vi "Find Post-Setup Actors.vi"(11 "Base Actor in":refnum<class "Base Actor.lvclass">) -> (2 "Post-Setup Actors":refnum<class "Actor.lvclass">[](array[class]))   [LabVIEW 2020, in "jettl.lvlib" / "Base jettl Actor.lvlib" / "Base Actor.lvlib" / "Base Actor.lvclass"]
uses:
  Base Actor.lvclass
  Base Actor.lvclass/Base Actor.ctl
  Actor/Actor.lvclass
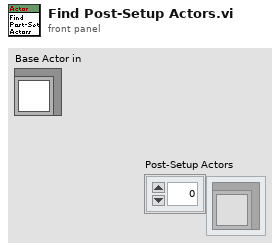
[diagram p1: front panel]
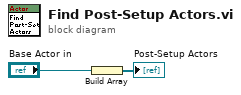
[diagram p0: block diagram]
diagram:
  n1 = Build Array("Base Actor in") -> (→"Post-Setup Actors":refnum<class "Base Actor.lvclass">[])
